vi "Update Display Objects.vi"(8 "Error In":errorcluster, 11 "Display Manager In":refnum<class "Display Manager.lvclass">) -> (0 "Error Out":errorcluster, 3 "Display Manager Out":refnum<class "Display Manager.lvclass">)   [LabVIEW 2019, in "Display Manager.lvclass"]
uses:
  Display Manager.lvclass
  Accessors/Display Mode/Get Display Mode.vi
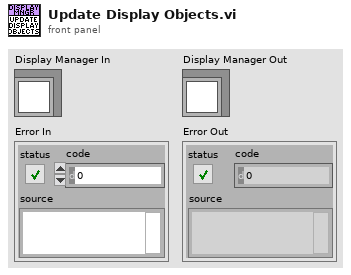
[diagram p1: front panel]
types:
  T1 = typedef "Display Manager.lvclass/Display Mode.ctl" = enum16{"Time", "Audio Analyzer", "Weather"}
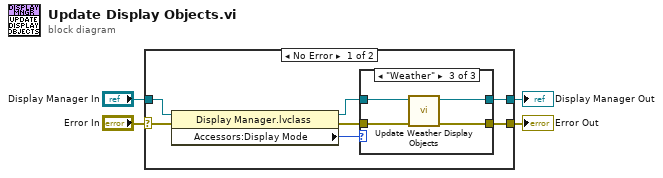
[diagram p0: block diagram]
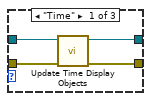
[diagram p2: hidden frame]
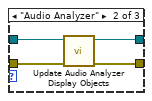
[diagram p3: hidden frame]
diagram:
  n1 = case shown="No Error" "Error In" {
    selector: "Error In" -> [w10 w25]
    tunnel: [w5 w25] -> w3
    tunnel: "Display Manager In" -> [w11 w24]
    tunnel: [w8 w24] -> w1
    frame No Error {
      n2 = property class="Display Manager.lvclass"(reference=w11, error in=w10) -> (reference out=w6:refnum<class "Display Manager.lvclass">, error out=w7:errorcluster, "Accessors:Display Mode"=w9:T1)
      n3 = case shown="\"Weather\"" w9 {
        tunnel: [w13 w17 w21] -> w8
        tunnel: w7 -> [w15 w19 w22]
        tunnel: w6 -> [w14 w18 w23]
        tunnel: [w12 w16 w20] -> w5
        frame "Time" {
          n4 = call "Update Time Display Objects.vi"("Error In"=w15, "Display Manager In"=w14) -> ("Error Out"=w12:errorcluster, "Display Manager Out"=w13:refnum<class "Display Manager.lvclass">)  [unwired: 8 in]
        }
        frame "Audio Analyzer" {
          n5 = call "Update Audio Analyzer Display Objects.vi"("Error In"=w19, "Display Manager In"=w18) -> ("Error Out"=w16:errorcluster, "Display Manager Out"=w17:refnum<class "Display Manager.lvclass">)  [unwired: 8 in]
        }
        frame "Weather" {
          n6 = call "Update Weather Display Objects.vi"("Error In"=w22, "Display Manager In"=w23) -> ("Error Out"=w20:errorcluster, "Display Manager Out"=w21:refnum<class "Display Manager.lvclass">)  [unwired: 8 in]
        }
      }
    }
    frame Error {
    }
  }
  "Display Manager Out" <- w1
  "Error Out" <- w3
